vi "Acquisition.vi"(8 "error in (no error)":errorcluster caption="entrée d'erreur (pas d'erreur)", 10 "Session In":T1, 11 "Acq Cam Basler en entrée":refnum<class "Acq Cam Basler.lvclass">) -> (0 "error out":errorcluster caption="sortie d'erreur", 2 "Session Out":T1, 3 "Acq Cam Basler en sortie":refnum<class "Acq Cam Basler.lvclass">)   [LabVIEW 2023, in "Acq Cam Basler.lvclass"]
uses:
  Acq Cam Basler.lvclass
  <vilib>/userDefined/High Color/IMAQdx.ctl
  <vilib>/vision/driver/IMAQdx.llb/IMAQdx Buffer Number Mode.ctl
  UI Cam Basler/Data Image.ctl
  <vilib>/vision/Image Controls.llb/IMAQ Image.ctl
  Acq Cam Basler.lvclass/Acq Cam Basler.ctl
  <vilib>/vision/driver/NI_Vision_Acquisition_Software.lvlib
  UI Cam Basler/UI Cam Basler.lvclass
panel:
  out "Image":T2(plugin-control)
  out "Images Missed":u32
  out "Processing Frame Rate":dbl
  out "Images Behind":i32
  out "Buffer Number":u32
  out "Acquired Frame Rate":dbl
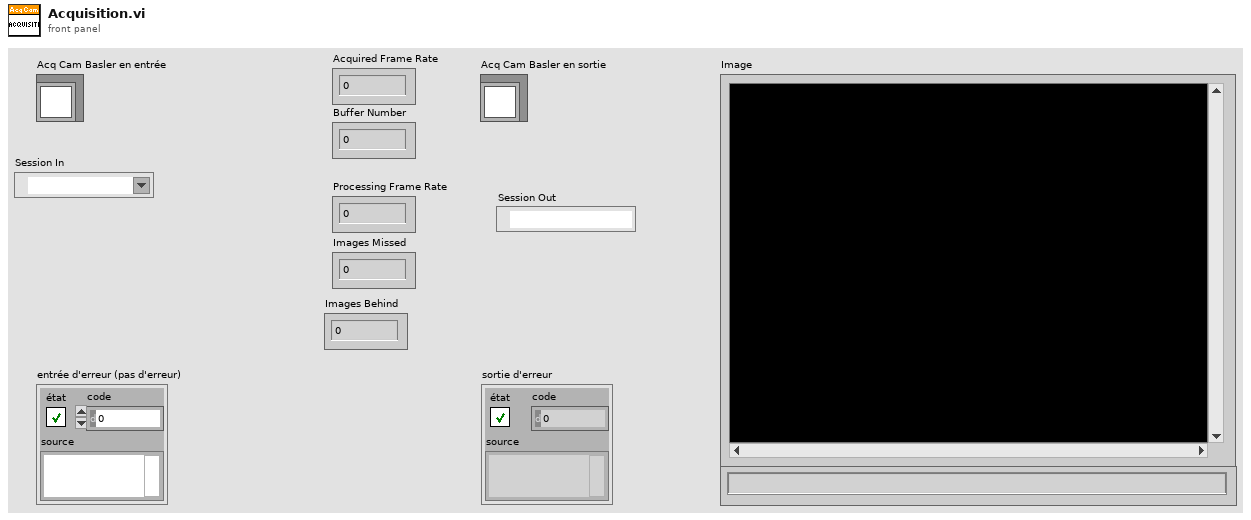
[diagram p1: front panel]
types:
  T1 = typedef "IMAQdx.ctl" = refnum<k21>
  T2 = typedef "IMAQ Image.ctl" = refnum<image>
  T3 = typedef "UI Cam Basler.lvclass/Data Image.ctl" = cluster{"Image Out":T2, "FPS":dbl}
  T4 = typedef "NI_Vision_Acquisition_Software.lvlib/IMAQdx Buffer Number Mode.ctl" = enum32{"Next", "Last", "Buffer Number", "Every", "Last New"}
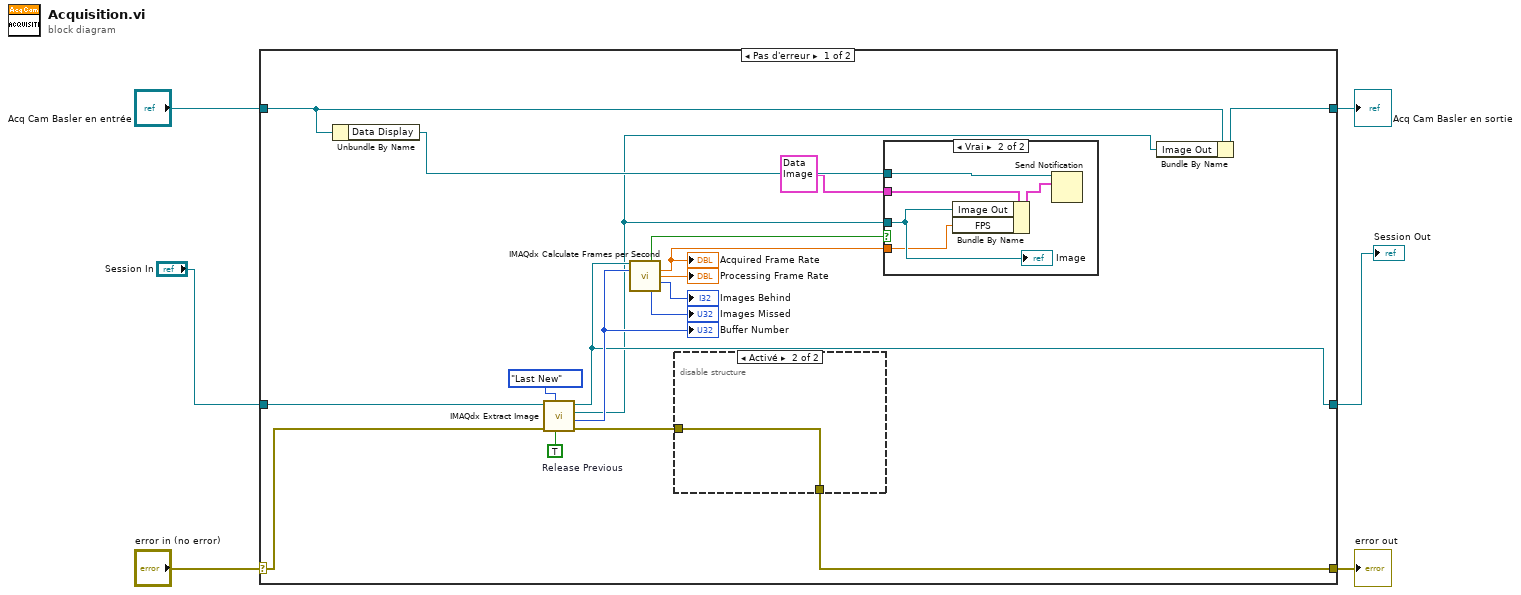
[diagram p0: block diagram]
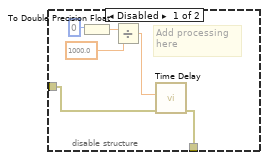
[diagram p2: hidden frame]
diagram:
  n1 = case shown="Pas d'erreur" "error in (no error)" {
    selector: "error in (no error)" -> [w15 w39]
    tunnel: [w14 w39] -> w5
    tunnel: [w12 w38] -> w3
    tunnel: "Acq Cam Basler en entrée" -> [w11 w38]
    tunnel: "Session In" -> [w16 w37]
    tunnel: [w13 w37] -> w1
    frame No Error {
      w23 = TRUE  # Release Previous
      n2 = Unbundle By Name(w11) -> ("Data Display"=w10:refnum<notifier>)
      n3 = call <vilib>:"IMAQdx Extract Image.vi"("Release Previous (true)"=w23, "Buffer Number Mode (Next)"=IMAQdx_Buffer_Number_Mode."Last New" ("Buffer Number Mode"), "error in"=w15, "Session In"=w16) -> ("error out"=w19:errorcluster, "Buffer Number Out"=w22:u32, "Image Out"=w7:T2, "Session Out"=w13:T1)  [unwired: 4 in]
      "Buffer Number" <- w22
      n4 = call <vilib>:"IMAQdx Calculate Frames per Second.vi"("Session In"=w13, "Buffer Number"=w22) -> ("Update Display"=w20:bool, "Acquired Frames per Second"=w8:dbl, "Processed Frames per Second"=→"Processing Frame Rate":dbl, "Images Behind"=→"Images Behind":i32, "Images Missed"=→"Images Missed":u32)  [unwired: 7 in, 2 out]
      "Acquired Frame Rate" <- w8
      n5 = disable-structure shown="Activé" {
        disable-tunnel: w19 -> [w30 w31]
        disable-tunnel: [w25 w31] -> w14
        frame Disabled {
          # "Add processing here"
          n6 = To Double Precision Float(number=0 ("Simulated Processing Delay (ms)")) -> (double precision float=w26:dbl)
          n7 = Divide(x=w26, y=1000.0) -> (x/y=w27:dbl)
          n8 = call "Time Delay"("error in (no error)"=w30, "Delay Time (s)"=w27) -> ("error out"=w25:errorcluster)  [unwired: 9 in]
        }
        frame Enabled {
        }
      }
      n9 = case shown="Vrai" w20 {
        tunnel: w7 -> [_ w33]
        tunnel: w10 -> [_ w36]
        tunnel: T3 {"Image Out"=refnum, "FPS"=0.0} ("notification") -> [_ w35]
        tunnel: w8 -> [_ w32]
        frame False {
        }
        frame True {
          n10 = Bundle By Name(cluster=w35, "Image Out"=w33, "FPS"=w32) -> (w34:T3)
          n11 = Send Notification(notification=w34, notifier=w36) -> ()  [unwired: 1 in, 2 out]
          "Image" <- w33
        }
      }
      n12 = Bundle By Name(cluster=w11, "Image Out"=w7) -> (w12:refnum<class "Acq Cam Basler.lvclass">)
    }
    frame Error {
    }
  }
  "error out" <- w5
  "Acq Cam Basler en sortie" <- w3
  "Session Out" <- w1
